vi "Tbl2Array.vi"(11 "strTable":string[][](table)) -> (3 "dblArray":dbl[][](array[numeric]))   [LabVIEW 2014, in "WfrmPlugins.lvlib" / "BaseWfrmPlugin.lvclass"]
uses:
  BaseWfrmPlugin.lvclass
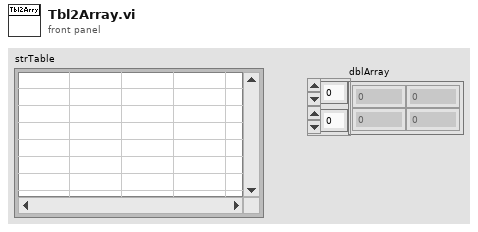
[diagram p1: front panel]
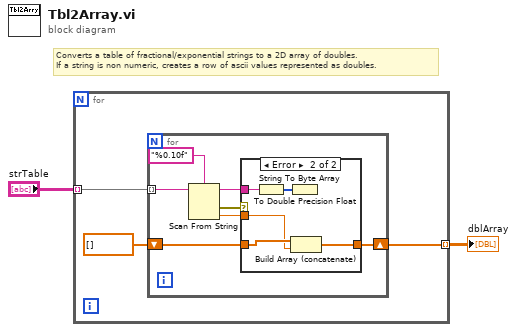
[diagram p0: block diagram]
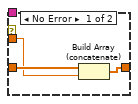
[diagram p2: hidden frame]
diagram:
  # "Converts a table of fractional/exponential strings to a 2D array of doubles.\nIf a string is non numeric, creates a row of ascii values represented as doubles."
  n1 = for {
    tunnel: "strTable" -> [w5] mode=indexing
    tunnel: [w3] -> w1 mode=indexing
    n2 = for {
      tunnel: w5 -> [w11] mode=indexing
      shift-right: [w7] -> w3
      shift-left: dbl[] [] -> [w8]
      n3 = Scan From String(format string="%0.10f", input string=w11) -> (remaining string=w9:string, error out=w10:errorcluster, output 1=w6:dbl)  [unwired: 3 in, 1 out]
      n4 = case shown="Error" w10 {
        tunnel: w9 -> [_ w20]
        tunnel: w8 -> [w15 w17]
        tunnel: [w13 w18] -> w7
        tunnel: w6 -> [w14 w16]
        frame No Error {
          n5 = Build Array (concatenate)(w15, w14) -> (w13:dbl[])
        }
        frame Error {
          n6 = String To Byte Array(string=w20) -> (unsigned byte array=w19:u8[])
          n7 = To Double Precision Float(number=w19) -> ()  [unwired: 1 out]
          n8 = Build Array (concatenate)(w17, w16) -> (w18:dbl[])
        }
      }
    }
  }
  "dblArray" <- w1
